vi "NewGame.vi"(8 "error in (no error)":errorcluster, 10 "Engine in":refnum<class "Engine.lvclass">, 11 "PongDemoType (ChildObject)":refnum<class "PongDemo.lvclass">) -> (0 "error out":errorcluster, 2 "Engine out":refnum<class "Engine.lvclass">, 3 "PongDemo out":refnum<class "PongDemo.lvclass">)   [LabVIEW 2019, in "RT_Game.lvlib" / "PongDemo.lvclass"]
uses:
  PongDemo.lvclass
  C:/Users/FreshBob/Dropbox/VIs/myRIO_GameConsole/RT/RT_Game/Game/Game.lvclass
  Engine/Engine.lvclass
  Game/Game.lvclass/Game.ctl
  Game/Write HasHighscore_.vi
  Game/Write HasMenu_.vi
  Pong/Pong.lvclass
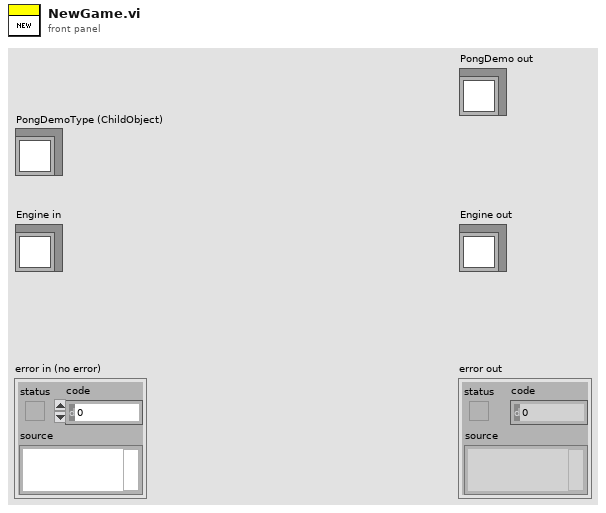
[diagram p1: front panel]
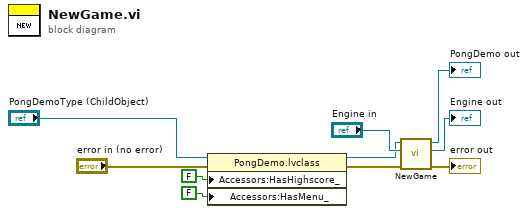
[diagram p0: block diagram]
diagram:
  n1 = property class="PongDemo.lvclass"(reference="PongDemoType (ChildObject)", error in="error in (no error)", "Accessors:HasHighscore_"=FALSE ("HasHighscore_"), "Accessors:HasMenu_"=FALSE ("HasMenu_")) -> (reference out=w3:refnum<class "PongDemo.lvclass">, error out=w5:errorcluster)
  n2 = call-parent "NewGame.vi"("error in (no error)"=w5, "Engine in"="Engine in", "PongType (ChildObject)"=w3) -> ("error out"=→"error out":errorcluster, "Engine out"=→"Engine out":refnum<class "Engine.lvclass">, "Pong out"=→"PongDemo out":refnum<class "PongDemo.lvclass">)  [unwired: 6 in]
